vi "Read Write App Config.vi"(7 "Write (F)":bool, 8 "Error IN":errorcluster, 10 "App Config IN":T1, 11 "Refnum in":T3) -> (0 "Error OUT":errorcluster, 2 "App Config OUT":T1, 3 "Refnum out":T3)   [LabVIEW 2013]
uses:
  <vilib>/Utility/config.llb/Config Data RefNum.ctl
  Type Defs/App Config.ctl
  Type Defs/Controller Names.ctl
  <vilib>/Utility/config.llb/Write Key (String).vi
  <vilib>/Utility/config.llb/Write Key (Path).vi
  <vilib>/Utility/config.llb/Write Key (U32).vi
  <vilib>/Utility/config.llb/Write Key (Double).vi
  <vilib>/Utility/config.llb/Write Key (I32).vi
  <vilib>/Utility/config.llb/Write Key (Boolean).vi
  <vilib>/Utility/config.llb/Read Key (String).vi
  <vilib>/Utility/config.llb/Read Key (Path).vi
  <vilib>/Utility/config.llb/Read Key (U32).vi
  <vilib>/Utility/config.llb/Read Key (Double).vi
  <vilib>/Utility/config.llb/Read Key (I32).vi
  <vilib>/Utility/config.llb/Read Key (Boolean).vi
  <vilib>/Utility/config.llb/NI_LVConfig.lvlib
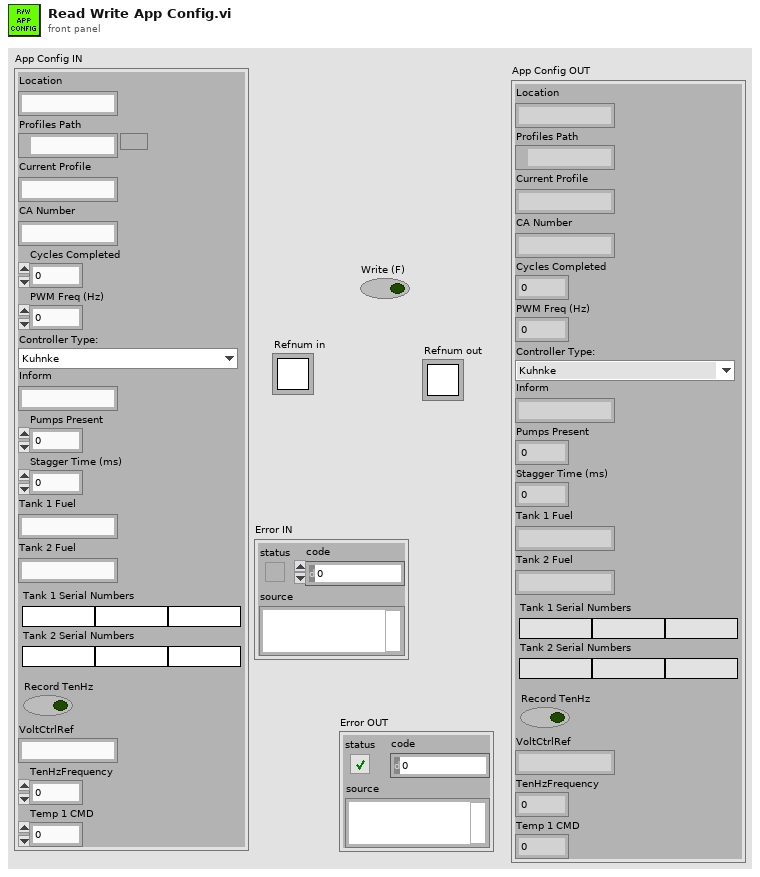
[diagram p1: front panel]
types:
  T1 = typedef "App Config.ctl" = cluster{"Location":string, "Profiles Path":path, "Current Profile":string, "CA Number":string, "Cycles Completed":u32, "PWM Freq (Hz)":dbl, "Controller Type:":T2, "Inform":string, "Pumps Present":u32, "Stagger Time (ms)":i32, "Tank 1 Fuel":string, "Tank 2 Fuel":string, "Serial Numbers":cluster{"Position 1 SN":string, "Position 2 SN":string, "Poaition 3 SN":string, "Position 4 SN":string, "Position 5 SN":string, "Position 6 SN":string}, "Record TenHz":bool, "VoltCtrlRef":string, "TenHzFrequency":u32, "Temp 1 CMD":dbl}
  T2 = typedef "Controller Names.ctl" = enum16{"Kuhnke", "Conti", "Hella CAN", "Helbako", "TI PWM", "PSA", "Hella DC Gas", "Hella DC Diesel", "8 Comm", "10 Comm", "8 Comm Hella", "10 Comm Hella", "8 Comm Omron", "10 Comm Omron", "8 Comm Nissan", "10 Comm Nissan"}
  T3 = typedef "NI_LVConfig.lvlib/Config Data RefNum.ctl" = refnum<k1>
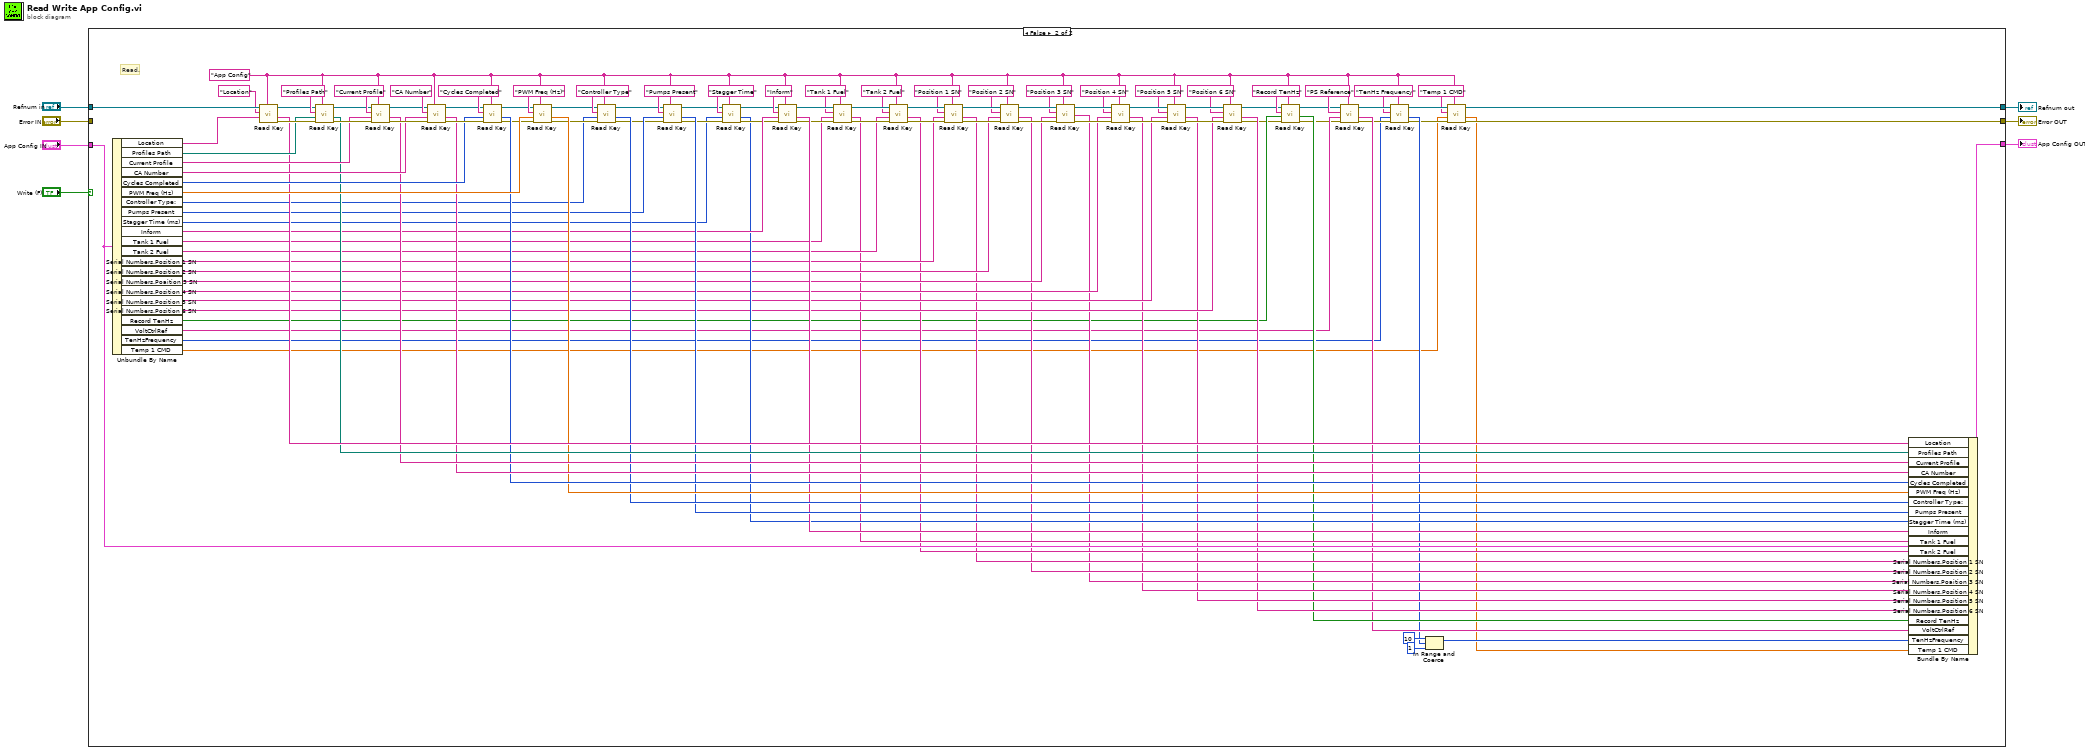
[diagram p0: block diagram]
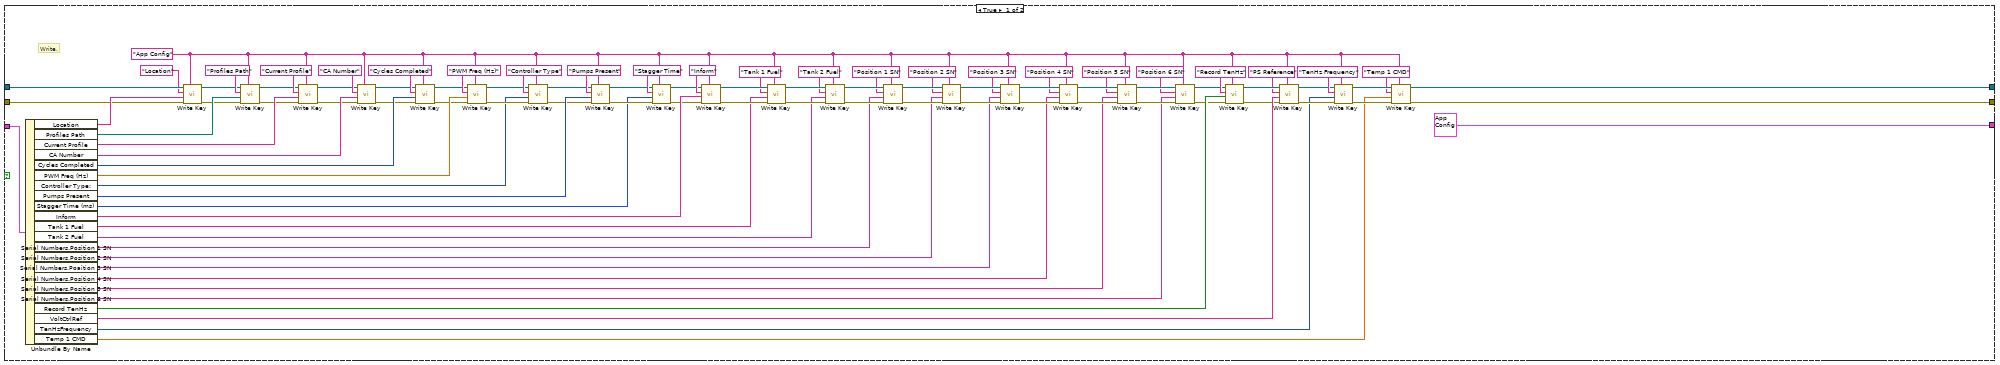
[diagram p2: hidden frame]
diagram:
  n1 = case shown="False" "Write (F)" {
    tunnel: "App Config IN" -> [w100 w169]
    tunnel: "Refnum in" -> [w99 w217]
    tunnel: [w12 w106] -> w4
    tunnel: [w11 w105] -> w3
    tunnel: [T1 {"Location"="", "Profiles Path"=path "", "Current Profile"="", "CA Number"="", "Cycles Completed"=0, "PWM Freq (Hz)"=0.0, "Controller Type:"=enum."Kuhnke", "Inform"="", "Pumps Present"=0, "Stagger Time (ms)"=0, "Tank 1 Fuel"="", "Tank 2 Fuel"="", "Serial Numbers"={"Position 1 SN"="", "Position 2 SN"="", "Poaition 3 SN"="", "Position 4 SN"="", "Position 5 SN"="", "Position 6 SN"=""}, "Record TenHz"=FALSE, "VoltCtrlRef"="", "TenHzFrequency"=0, "Temp 1 CMD"=0.0} ("App Config IN") w168] -> w2
    tunnel: "Error IN" -> [w77 _]
    frame True {
      w10 = "App Config" ("section")
      # "Write."
      n2 = Unbundle By Name(w100) -> ("Location"=w97:string, "Profiles Path"=w91:path, "Current Profile"=w90:string, "CA Number"=w89:string, "Cycles Completed"=w88:u32, "PWM Freq (Hz)"=w87:dbl, "Controller Type:"=w74:T2, "Pumps Present"=w69:u32, "Stagger Time (ms)"=w59:i32, "Inform"=w65:string, "Tank 1 Fuel"=w42:string, "Tank 2 Fuel"=w41:string, "Serial Numbers.Position 1 SN"=w40:string, "Serial Numbers.Position 2 SN"=w39:string, "Serial Numbers.Poaition 3 SN"=w38:string, "Serial Numbers.Position 4 SN"=w37:string, "Serial Numbers.Position 5 SN"=w36:string, "Serial Numbers.Position 6 SN"=w35:string, "Record TenHz"=w25:bool, "VoltCtrlRef"=w24:string, "TenHzFrequency"=w17:u32, "Temp 1 CMD"=w8:dbl)
      n3 = call-poly <vilib>:"Write Key.vi"("section"=w10, "error in (no error)"=w77, "value"=w97, "key"="Location" ("section"), "refnum"=w99) -> ("error out"=w86:errorcluster, "refnum out"=w85:T3)  [unwired: 4 in, 1 out]
      n4 = call-poly <vilib>:"Write Key.vi"("section"=w10, "error in (no error)"=w86, "value"=w91, "key"="Profiles Path" ("section"), "refnum"=w85) -> ("error out"=w83:errorcluster, "refnum out"=w84:T3)  [unwired: 4 in, 1 out]
      n5 = call-poly <vilib>:"Write Key.vi"("section"=w10, "error in (no error)"=w83, "value"=w90, "key"="Current Profile" ("section"), "refnum"=w84) -> ("error out"=w81:errorcluster, "refnum out"=w82:T3)  [unwired: 4 in, 1 out]
      n6 = call-poly <vilib>:"Write Key.vi"("section"=w10, "error in (no error)"=w81, "value"=w89, "key"="CA Number" ("section"), "refnum"=w82) -> ("error out"=w79:errorcluster, "refnum out"=w80:T3)  [unwired: 4 in, 1 out]
      n7 = call-poly <vilib>:"Write Key.vi"("section"=w10, "error in (no error)"=w79, "value"=w88, "key"="Cycles Completed" ("section"), "refnum"=w80) -> ("error out"=w71:errorcluster, "refnum out"=w72:T3)  [unwired: 4 in, 1 out]
      n8 = call-poly <vilib>:"Write Key.vi"("section"=w10, "error in (no error)"=w71, "value"=w87, "key"="PWM Freq (Hz)" ("section"), "refnum"=w72) -> ("error out"=w75:errorcluster, "refnum out"=w73:T3)  [unwired: 4 in, 1 out]
      n9 = call-poly <vilib>:"Write Key.vi"("section"=w10, "error in (no error)"=w75, "value"=w74, "key"="Controller Type" ("section"), "refnum"=w73) -> ("error out"=w67:errorcluster, "refnum out"=w68:T3)  [unwired: 4 in, 1 out]
      n10 = call-poly <vilib>:"Write Key.vi"("section"=w10, "error in (no error)"=w67, "value"=w69, "key"="Pumps Present" ("section"), "refnum"=w68) -> ("error out"=w62:errorcluster, "refnum out"=w63:T3)  [unwired: 4 in, 1 out]
      n11 = call-poly <vilib>:"Write Key.vi"("section"=w10, "error in (no error)"=w62, "value"=w59, "key"="Stagger Time" ("section"), "refnum"=w63) -> ("error out"=w61:errorcluster, "refnum out"=w60:T3)  [unwired: 4 in, 1 out]
      n12 = call-poly <vilib>:"Write Key.vi"("section"=w10, "error in (no error)"=w61, "value"=w65, "key"="Inform" ("section"), "refnum"=w60) -> ("error out"=w43:errorcluster, "refnum out"=w58:T3)  [unwired: 4 in, 1 out]
      n13 = call-poly <vilib>:"Write Key.vi"("section"=w10, "error in (no error)"=w43, "value"=w42, "key"="Tank 1 Fuel", "refnum"=w58) -> ("error out"=w44:errorcluster, "refnum out"=w57:T3)  [unwired: 4 in, 1 out]
      n14 = call-poly <vilib>:"Write Key.vi"("section"=w10, "error in (no error)"=w44, "value"=w41, "key"="Tank 2 Fuel", "refnum"=w57) -> ("error out"=w45:errorcluster, "refnum out"=w56:T3)  [unwired: 4 in, 1 out]
      n15 = call-poly <vilib>:"Write Key.vi"("section"=w10, "error in (no error)"=w45, "value"=w40, "key"="Position 1 SN", "refnum"=w56) -> ("error out"=w46:errorcluster, "refnum out"=w55:T3)  [unwired: 4 in, 1 out]
      n16 = call-poly <vilib>:"Write Key.vi"("section"=w10, "error in (no error)"=w46, "value"=w39, "key"="Position 2 SN", "refnum"=w55) -> ("error out"=w47:errorcluster, "refnum out"=w54:T3)  [unwired: 4 in, 1 out]
      n17 = call-poly <vilib>:"Write Key.vi"("section"=w10, "error in (no error)"=w47, "value"=w38, "key"="Position 3 SN", "refnum"=w54) -> ("error out"=w48:errorcluster, "refnum out"=w53:T3)  [unwired: 4 in, 1 out]
      n18 = call-poly <vilib>:"Write Key.vi"("section"=w10, "error in (no error)"=w48, "value"=w37, "key"="Position 4 SN", "refnum"=w53) -> ("error out"=w49:errorcluster, "refnum out"=w52:T3)  [unwired: 4 in, 1 out]
      n19 = call-poly <vilib>:"Write Key.vi"("section"=w10, "error in (no error)"=w49, "value"=w36, "key"="Position 5 SN", "refnum"=w52) -> ("error out"=w50:errorcluster, "refnum out"=w51:T3)  [unwired: 4 in, 1 out]
      n20 = call-poly <vilib>:"Write Key.vi"("section"=w10, "error in (no error)"=w50, "value"=w35, "key"="Position 6 SN", "refnum"=w51) -> ("error out"=w15:errorcluster, "refnum out"=w16:T3)  [unwired: 4 in, 1 out]
      n21 = call-poly <vilib>:"Write Key.vi"("section"=w10, "error in (no error)"=w15, "value"=w25, "key"="Record TenHz", "refnum"=w16) -> ("error out"=w23:errorcluster, "refnum out"=w22:T3)  [unwired: 4 in, 1 out]
      n22 = call-poly <vilib>:"Write Key.vi"("section"=w10, "error in (no error)"=w23, "value"=w24, "key"="PS Reference", "refnum"=w22) -> ("error out"=w19:errorcluster, "refnum out"=w18:T3)  [unwired: 4 in, 1 out]
      n23 = call-poly <vilib>:"Write Key.vi"("section"=w10, "error in (no error)"=w19, "value"=w17, "key"="TenHz Frequency", "refnum"=w18) -> ("error out"=w13:errorcluster, "refnum out"=w14:T3)  [unwired: 4 in, 1 out]
      n24 = call-poly <vilib>:"Write Key.vi"("section"=w10, "error in (no error)"=w13, "value"=w8, "key"="Temp 1 CMD", "refnum"=w14) -> ("error out"=w11:errorcluster, "refnum out"=w12:T3)  [unwired: 4 in, 1 out]
    }
    frame False {
      w104 = "App Config" ("section")
      # "Read."
      n25 = Unbundle By Name(w169) -> ("Location"=w202:string, "Profiles Path"=w201:path, "Current Profile"=w200:string, "CA Number"=w199:string, "Cycles Completed"=w198:u32, "PWM Freq (Hz)"=w197:dbl, "Controller Type:"=w115:T2, "Pumps Present"=w183:u32, "Stagger Time (ms)"=w171:i32, "Inform"=w178:string, "Tank 1 Fuel"=w143:string, "Tank 2 Fuel"=w142:string, "Serial Numbers.Position 1 SN"=w141:string, "Serial Numbers.Position 2 SN"=w140:string, "Serial Numbers.Poaition 3 SN"=w139:string, "Serial Numbers.Position 4 SN"=w138:string, "Serial Numbers.Position 5 SN"=w137:string, "Serial Numbers.Position 6 SN"=w136:string, "Record TenHz"=w126:bool, "VoltCtrlRef"=w123:string, "TenHzFrequency"=w117:u32, "Temp 1 CMD"=w102:dbl)
      n26 = call-poly <vilib>:"Read Key.vi"("section"=w104, "default value"=w202, "key"="Location" ("section"), "refnum"=w217) -> ("error out"=w210:errorcluster, "value"=w196:string, "refnum out"=w209:T3)  [unwired: 4 in, 1 out]
      n27 = call-poly <vilib>:"Read Key.vi"("section"=w104, "error in (no error)"=w210, "default value"=w201, "key"="Profiles Path" ("section"), "refnum"=w209) -> ("error out"=w207:errorcluster, "value"=w195:path, "refnum out"=w208:T3)  [unwired: 3 in, 1 out]
      n28 = call-poly <vilib>:"Read Key.vi"("section"=w104, "error in (no error)"=w207, "default value"=w200, "key"="Current Profile" ("section"), "refnum"=w208) -> ("error out"=w205:errorcluster, "value"=w194:string, "refnum out"=w206:T3)  [unwired: 3 in, 1 out]
      n29 = call-poly <vilib>:"Read Key.vi"("section"=w104, "error in (no error)"=w205, "default value"=w199, "key"="CA Number" ("section"), "refnum"=w206) -> ("error out"=w203:errorcluster, "value"=w193:string, "refnum out"=w204:T3)  [unwired: 3 in, 1 out]
      n30 = call-poly <vilib>:"Read Key.vi"("section"=w104, "error in (no error)"=w203, "default value"=w198, "key"="Cycles Completed" ("section"), "refnum"=w204) -> ("error out"=w185:errorcluster, "value"=w192:u32, "refnum out"=w186:T3)  [unwired: 3 in, 1 out]
      n31 = call-poly <vilib>:"Read Key.vi"("section"=w104, "error in (no error)"=w185, "default value"=w197, "key"="PWM Freq (Hz)" ("section"), "refnum"=w186) -> ("error out"=w188:errorcluster, "value"=w191:dbl, "refnum out"=w189:T3)  [unwired: 3 in, 1 out]
      n32 = call-poly <vilib>:"Read Key.vi"("section"=w104, "error in (no error)"=w188, "default value"=w115, "key"="Controller Type" ("section"), "refnum"=w189) -> ("error out"=w182:errorcluster, "value"=w187:i32, "refnum out"=w181:T3)  [unwired: 3 in, 1 out]
      n33 = call-poly <vilib>:"Read Key.vi"("section"=w104, "error in (no error)"=w182, "default value"=w183, "key"="Pumps Present" ("section"), "refnum"=w181) -> ("error out"=w175:errorcluster, "value"=w180:u32, "refnum out"=w174:T3)  [unwired: 3 in, 1 out]
      n34 = call-poly <vilib>:"Read Key.vi"("section"=w104, "error in (no error)"=w175, "default value"=w171, "key"="Stagger Time" ("section"), "refnum"=w174) -> ("error out"=w172:errorcluster, "value"=w170:i32, "refnum out"=w173:T3)  [unwired: 3 in, 1 out]
      n35 = call-poly <vilib>:"Read Key.vi"("section"=w104, "error in (no error)"=w172, "default value"=w178, "key"="Inform" ("section"), "refnum"=w173) -> ("error out"=w159:errorcluster, "value"=w177:string, "refnum out"=w167:T3)  [unwired: 3 in, 1 out]
      n36 = call-poly <vilib>:"Read Key.vi"("section"=w104, "error in (no error)"=w159, "default value"=w143, "key"="Tank 1 Fuel", "refnum"=w167) -> ("error out"=w158:errorcluster, "value"=w135:string, "refnum out"=w166:T3)  [unwired: 3 in, 1 out]
      n37 = call-poly <vilib>:"Read Key.vi"("section"=w104, "error in (no error)"=w158, "default value"=w142, "key"="Tank 2 Fuel", "refnum"=w166) -> ("error out"=w157:errorcluster, "value"=w134:string, "refnum out"=w165:T3)  [unwired: 3 in, 1 out]
      n38 = call-poly <vilib>:"Read Key.vi"("section"=w104, "error in (no error)"=w157, "default value"=w141, "key"="Position 1 SN", "refnum"=w165) -> ("error out"=w156:errorcluster, "value"=w133:string, "refnum out"=w164:T3)  [unwired: 3 in, 1 out]
      n39 = call-poly <vilib>:"Read Key.vi"("section"=w104, "error in (no error)"=w156, "default value"=w140, "key"="Position 2 SN", "refnum"=w164) -> ("error out"=w155:errorcluster, "value"=w132:string, "refnum out"=w163:T3)  [unwired: 3 in, 1 out]
      n40 = call-poly <vilib>:"Read Key.vi"("section"=w104, "error in (no error)"=w155, "default value"=w139, "key"="Position 3 SN", "refnum"=w163) -> ("error out"=w154:errorcluster, "value"=w131:string, "refnum out"=w162:T3)  [unwired: 3 in, 1 out]
      n41 = call-poly <vilib>:"Read Key.vi"("section"=w104, "error in (no error)"=w154, "default value"=w138, "key"="Position 4 SN", "refnum"=w162) -> ("error out"=w153:errorcluster, "value"=w130:string, "refnum out"=w161:T3)  [unwired: 3 in, 1 out]
      n42 = call-poly <vilib>:"Read Key.vi"("section"=w104, "error in (no error)"=w153, "default value"=w137, "key"="Position 5 SN", "refnum"=w161) -> ("error out"=w152:errorcluster, "value"=w129:string, "refnum out"=w160:T3)  [unwired: 3 in, 1 out]
      n43 = call-poly <vilib>:"Read Key.vi"("section"=w104, "error in (no error)"=w152, "default value"=w136, "key"="Position 6 SN", "refnum"=w160) -> ("error out"=w109:errorcluster, "value"=w128:string, "refnum out"=w110:T3)  [unwired: 3 in, 1 out]
      n44 = call-poly <vilib>:"Read Key.vi"("section"=w104, "error in (no error)"=w109, "default value"=w126, "key"="Record TenHz", "refnum"=w110) -> ("error out"=w122:errorcluster, "value"=w125:bool, "refnum out"=w121:T3)  [unwired: 3 in, 1 out]
      n45 = call-poly <vilib>:"Read Key.vi"("section"=w104, "error in (no error)"=w122, "default value"=w123, "key"="PS Reference", "refnum"=w121) -> ("error out"=w118:errorcluster, "value"=w120:string, "refnum out"=w119:T3)  [unwired: 3 in, 1 out]
      n46 = call-poly <vilib>:"Read Key.vi"("section"=w104, "error in (no error)"=w118, "default value"=w117, "key"="TenHz Frequency", "refnum"=w119) -> ("error out"=w107:errorcluster, "value"=w112:u32, "refnum out"=w108:T3)  [unwired: 3 in, 1 out]
      n47 = In Range and Coerce(upper limit=u32 10, x=w112, lower limit=u32 1) -> (coerced(x)=w111:u32)  [unwired: 1 out]
      n48 = call-poly <vilib>:"Read Key.vi"("section"=w104, "error in (no error)"=w107, "default value"=w102, "key"="Temp 1 CMD", "refnum"=w108) -> ("error out"=w105:errorcluster, "value"=w101:dbl, "refnum out"=w106:T3)  [unwired: 3 in, 1 out]
      n49 = Bundle By Name(cluster=w169, "Location"=w196, "Profiles Path"=w195, "Current Profile"=w194, "CA Number"=w193, "Cycles Completed"=w192, "PWM Freq (Hz)"=w191, "Controller Type:"=w187, "Pumps Present"=w180, "Stagger Time (ms)"=w170, "Inform"=w177, "Tank 1 Fuel"=w135, "Tank 2 Fuel"=w134, "Serial Numbers.Position 1 SN"=w133, "Serial Numbers.Position 2 SN"=w132, "Serial Numbers.Poaition 3 SN"=w131, "Serial Numbers.Position 4 SN"=w130, "Serial Numbers.Position 5 SN"=w129, "Serial Numbers.Position 6 SN"=w128, "Record TenHz"=w125, "VoltCtrlRef"=w120, "TenHzFrequency"=w111, "Temp 1 CMD"=w101) -> (w168:T1)
    }
  }
  "Error OUT" <- w3
  "Refnum out" <- w4
  "App Config OUT" <- w2
